vi "G#Object_SendUserEvent.vi"(0 "refererence in":refnum<class "G#Object.lvclass">, 1 "text":string, 2 "parameters":variant[](array[variant]), 5 "error in (no error)":errorcluster, 6 "call depth (1)":i32=1, 7 "send to Desktop Trace Execution? (F)":bool) -> (14 "reference  out":refnum<class "G#Object.lvclass">, 19 "error out":errorcluster)   [LabVIEW 2020, in "G#Object.lvclass"]
doc: "Adds an G# user event that will show up in the debugger trace as well."
uses:
  <vilib>/addons/_AddQ/G#Object/G#Object.lvclass
  <vilib>/addons/_AddQ/G#Object/utils/G#Object_EventType.ctl
  <vilib>/addons/_AddQ/G#Object/utils/G#Object_ObjectInfoType.ctl
  <vilib>/addons/_AddQ/G#Object/utils/G#Object_CreateMethod.ctl
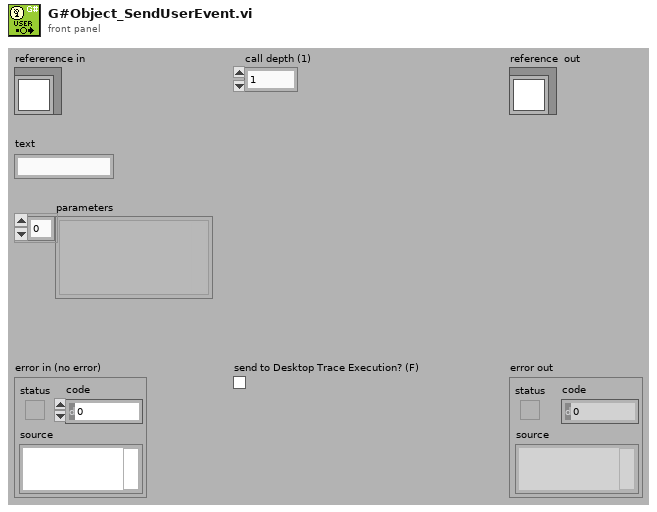
[diagram p1: front panel]
types:
  T1 = typedef "G#Object.lvclass/G#Object_ObjectInfoType.ctl" = cluster{"ObjectName":string, "ObjectID":u32, "Users":i32, "Counter":bool, "AttributeRefs":u32[], "FullClassName":string, "ClassName":string, "CreateMethod":T2, "GenericDestructorExists":bool, "Owner":string}
  T2 = typedef "G#Object.lvclass/G#Object_CreateMethod.ctl" = enum16{"Create", "Create or look up existing", "Look up existing"}
  T3 = typedef "G#Object.lvclass/G#Object_EventType.ctl" = enum16{"Created new", "Looked up existing", "Deleted", "Forced delete", "Not deleted", "Garbage collected", "Cleared", "User", "Error", "External create object", "External create class attributes", "Created class attributes", "Run constructor", "Run constructor done", "Run open method", "Run open method done"}
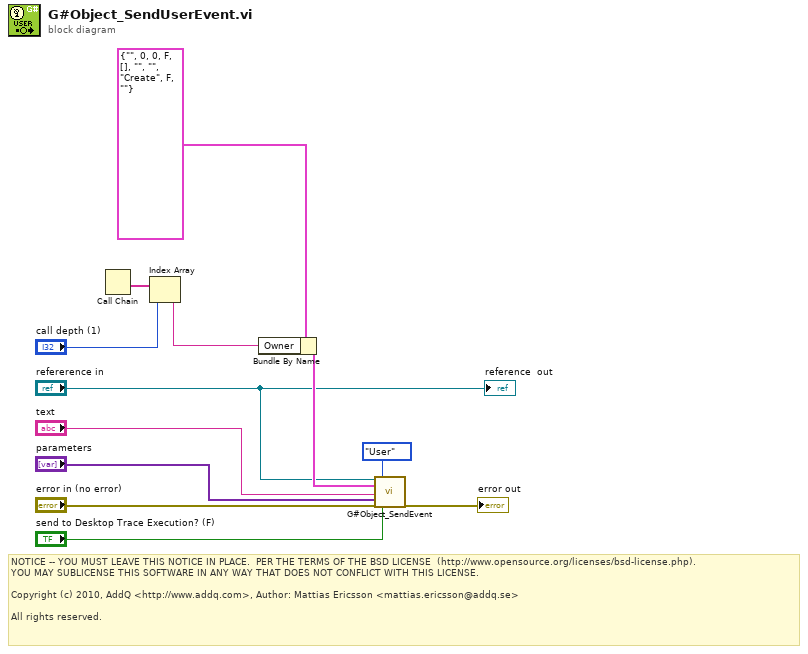
[diagram p0: block diagram]
diagram:
  # "NOTICE -- YOU MUST LEAVE THIS NOTICE IN PLACE.  PER THE TERMS OF THE BSD LICENSE  (http://www.opensource.org/licenses/bsd-license.php).\nYOU MAY SUBLICENSE THIS SOFTWARE IN ANY WAY THAT DOES NOT CONFLICT WITH THIS LICENSE.\n\nCopyright (c) 2010, AddQ <http://www.addq.com>, Author: Mattias Ericsson <mattias.ericsson@addq.se>\n\nAll rights reserved."
  n1 = Call Chain() -> (call chain=w4:string[])
  n2 = Index Array(array=w4, index="call depth (1)") -> (element=w2:string)
  n3 = Bundle By Name(cluster=T1 {"ObjectName"="", "ObjectID"=0, "Users"=0, "Counter"=FALSE, "AttributeRefs"=[], "FullClassName"="", "ClassName"="", "CreateMethod"=enum."Create", "GenericDestructorExists"=FALSE, "Owner"=""} ("object info extended"), "Owner"=w2) -> (w5:T1)
  n4 = call <vilib>:"G#Object_SendEvent.vi"("reference in"="refererence in", "object info extended"=w5, "comment"="text", "parameters"="parameters", "error in (no error)"="error in (no error)", "G# event type"=G#Object_EventType."User" ("G#Event"), "send to Desktop Trace Execution"="send to Desktop Trace Execution? (F)") -> ("error out"=→"error out":errorcluster)  [unwired: 12 in]
  "reference  out" <- "refererence in"
